vi "写入当前数据是否完成状态.vi"(8 "error in (no error)":errorcluster caption="错误输入（无错误）", 11 "抽取参数输入":refnum<class "抽取参数.lvclass">) -> (0 "error out":errorcluster caption="错误输出", 3 "抽取参数输出":refnum<class "抽取参数.lvclass">)   [LabVIEW 2020, in "抽取参数.lvclass"]
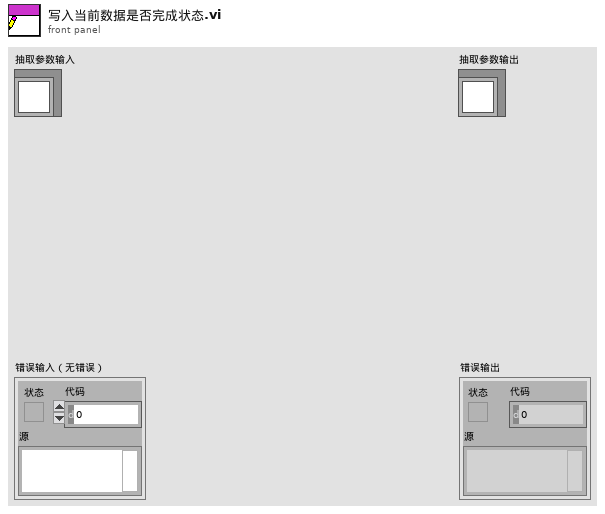
[diagram p1: front panel]
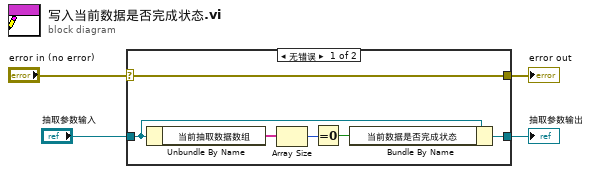
[diagram p0: block diagram]
diagram:
  n1 = case shown="无错误" "error in (no error)" {
    selector: "error in (no error)" -> [w10 w11]
    tunnel: [w10 w11] -> w3
    tunnel: [w9 w12] -> w1
    tunnel: "抽取参数输入" -> [w8 w12]
    frame No Error {
      n2 = Unbundle By Name(w8) -> ("当前抽取数据数组"=w7:string[])
      n3 = Array Size(array=w7) -> (size(s)=w6:i32)
      n4 = Equal To 0?(x=w6) -> (x = 0?=w5:bool)
      n5 = Bundle By Name(cluster=w8, "当前数据是否完成状态"=w5) -> (w9:refnum<class "抽取参数.lvclass">)
    }
    frame Error {
    }
  }
  "error out" <- w3
  "抽取参数输出" <- w1
